vi "Cyclic Frame Scheduler.vi"(9 "pending frames":u32[](array[numeric]), 10 "frame schedule":T1 {"Arb ID" format="%.0x"}, 11 "command":T2) -> (1 "frames to generate":u32[](array[numeric]))   [LabVIEW 2013, in "J1939.lvlib"]
uses:
  J1939.lvlib
  Cyclic Frame Scheduler LUT Command.ctl
  API Types/Periodic Message Generator Cluster.ctl
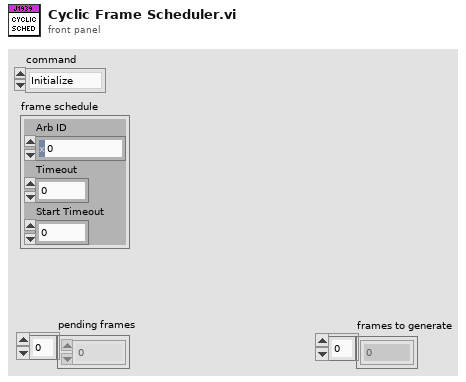
[diagram p1: front panel]
types:
  T1 = typedef "J1939.lvlib/Periodic Message Generator Cluster.ctl" = cluster{"Arb ID":u32, "Timeout":u32, "Start Timeout":u32}
  T2 = typedef "J1939.lvlib/cyclic frame scheduler lut command.ctl" = enum16{"Initialize", "set", "remove", "calculate times"}
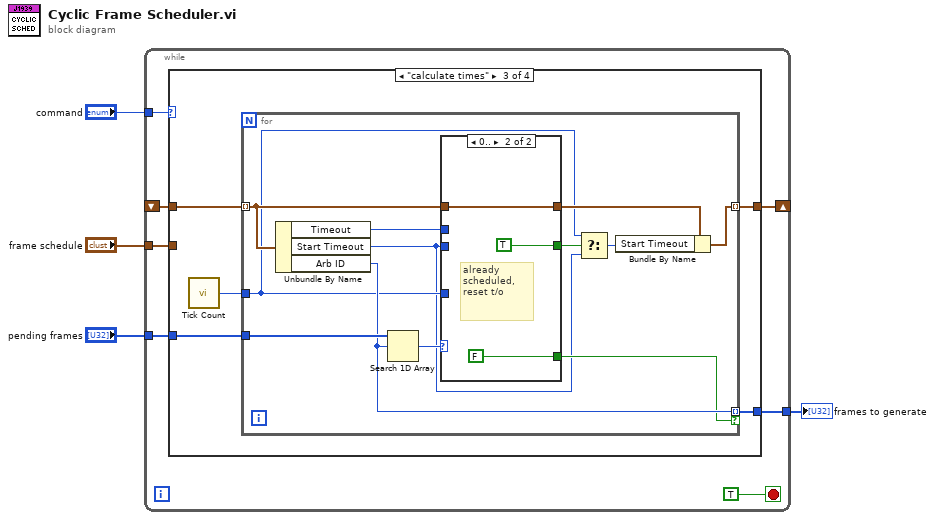
[diagram p0: block diagram]
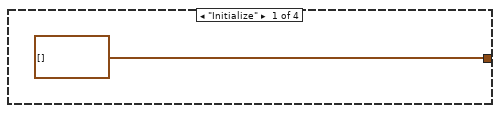
[diagram p2: hidden frame]
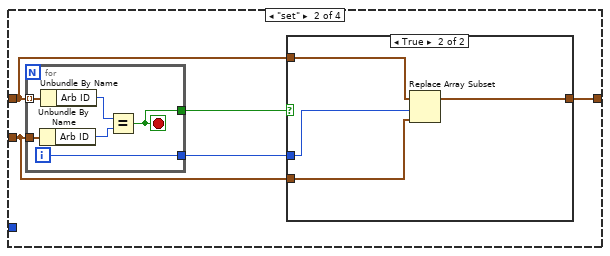
[diagram p3: hidden frame]
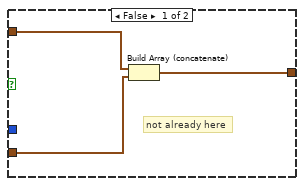
[diagram p4: hidden frame]
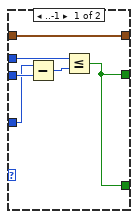
[diagram p5: hidden frame]
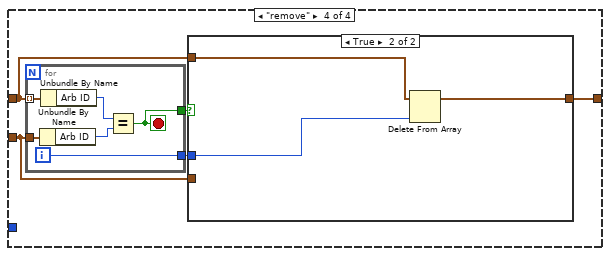
[diagram p6: hidden frame]
diagram:
  n1 = while {
    shift-right: [w9] -> _
    shift-left: _ -> [w10]
    tunnel: "command" -> [w11]
    tunnel: "frame schedule" -> [w7]
    tunnel: "pending frames" -> [w6]
    tunnel: [w5] -> w1
    stop <- TRUE stop-if-true
    n2 = case shown="\"calculate times\"" w11 {
      tunnel: w10 -> [_ w15 w34 w59]
      tunnel: [T1[] [] w14 w31 w58] -> w9
      tunnel: w7 -> [_ w13 _ w57]
      tunnel: w6 -> [_ _ w35 _]
      tunnel: [_ _ w32 _] -> w5
      frame "Initialize" {
      }
      frame "set" {
        n3 = for {
          tunnel: w15 -> [w30] mode=indexing
          tunnel: w13 -> [w28]
          tunnel: [w26] -> w16
          tunnel: [w25] -> w17
          i -> [w26]
          stop <- w25 stop-if-true
          n4 = Unbundle By Name(w28) -> ("Arb ID"=w27:u32)
          n5 = Unbundle By Name(w30) -> ("Arb ID"=w29:u32)
          n6 = Equal?(x=w29, y=w27) -> (x = y?=w25:bool)
        }
        n7 = case shown="True" w17 {
          tunnel: w16 -> [_ w22]
          tunnel: w15 -> [w19 w24]
          tunnel: [w18 w23] -> w14
          tunnel: w13 -> [w20 w21]
          frame False {
            # "not already here"
            n8 = Build Array (concatenate)(w19, w20) -> (w18:T1[])
          }
          frame True {
            n9 = Replace Array Subset(array=w24, new element=w21, index=w22) -> (w23:T1[])
          }
        }
      }
      frame "calculate times" {
        n10 = call "Tick Count"() -> ("Tick Count(mSec)"=w33:u32)
        n11 = for {
          tunnel: w35 -> [w47]
          tunnel: w34 -> [w43] mode=indexing
          tunnel: w33 -> [w38]
          tunnel: [w45] -> w32 mode=indexing if=w44
          tunnel: [w40] -> w31 mode=indexing
          n12 = Unbundle By Name(w43) -> ("Timeout"=w42:u32, "Start Timeout"=w37:u32, "Arb ID"=w45:u32)
          n13 = Search 1D Array(1D array=w47, element=w45) -> (index of element=w46:i32)  [unwired: 1 in]
          n14 = case shown="0.." w46 {
            tunnel: [w48 FALSE] -> w44
            tunnel: [w50 w55] -> w41
            tunnel: w43 -> [w50 w55]
            tunnel: w38 -> [w49 _]
            tunnel: w42 -> [w52 _]
            tunnel: w37 -> [w53 _]
            tunnel: [w48 TRUE] -> w39
            frame ..-1 {
              n15 = Subtract(x=w49, y=w53) -> (x-y=w51:u32)
              n16 = Less Or Equal?(x=w52, y=w51) -> (x <= y?=w48:bool)
            }
            frame 0.. {
              # "already scheduled, reset t/o"
            }
          }
          n17 = Select(t=w38, s=w39, f=w37) -> (s? t:f=w36:u32)
          n18 = Bundle By Name(cluster=w41, "Start Timeout"=w36) -> (w40:T1)
        }
      }
      frame "remove" {
        n19 = for {
          tunnel: w59 -> [w71] mode=indexing
          tunnel: w57 -> [w69]
          tunnel: [w67] -> w60
          tunnel: [w66] -> w61
          i -> [w67]
          stop <- w66 stop-if-true
          n20 = Unbundle By Name(w69) -> ("Arb ID"=w68:u32)
          n21 = Unbundle By Name(w71) -> ("Arb ID"=w70:u32)
          n22 = Equal?(x=w70, y=w68) -> (x = y?=w66:bool)
        }
        n23 = case shown="True" w61 {
          tunnel: w60 -> [_ w63]
          tunnel: w59 -> [w62 w65]
          tunnel: [w62 w64] -> w58
          tunnel: w57 -> [_ _]
          frame False {
            # "not here"
          }
          frame True {
            n24 = Delete From Array(array=w65, index=w63) -> (array with subset deleted=w64:T1[])  [unwired: 1 in, 1 out]
          }
        }
      }
    }
  }
  "frames to generate" <- w1
